vi "Gather_Deal_Data_BK.vi"(8 "strModelChoice":string(combo)="WD5500", 9 "写指令":bool=TRUE, 10 "VISA resource name":refnum<visa-resource-name>="COM1" caption="VISA资源名称") -> (2 "缓冲区数据":u32=284, 3 "strResultArrayOut":string[](array[string]))   [LabVIEW 2011]
uses:
  <vilib>/Instr/_visa.llb/VISA Configure Serial Port (Instr).vi
panel:
  out "mu08BufSize":u8
  out "mbfDealData":bool
  out "mu08SendCmd":u8=3
  in  "CmdNumCount":u8
  out "mu08ArrayBuf0":u8[](array[numeric])=[90, 165, 142, 1, 240, 0, 1, 88, 200, 2, 0, 207, 3, 0, 219, 7, 1, 40, 11, 0, 0, 12, 0, 0, 13, 0, 0, 14, 0, 0, 21, 0, 0, 22, 0, 0, 23, 0, 0, 24, 150, 154, 29, 0, 0, 0, 0, 31, 0, 0, 33, 0, 34, 1, 64, 35, 0, 41, 0, 42, 0, 43, 0, 44, 12, 158, 45, 0, 0, 46, 0, 240, 47, 240, 48, 0, 49, 0, 50, 136, 51, 0, 52, 0, 53, 0, 54, 132, 58, 0, 59, 0, 60, 241, 61, 32, 32, 32, 32, 82, 64, 73, 83, 90, 2, 4, 0, 2, 4, 0, 0, 0, 0, 2, 0, 0, 0, 104, 201, 113, 49, 49, 53, 202, 70, 52, 48, 53, 203, 57, 48, 48, 66, 204, 32, 32, 48, 53, 251, 6, 87, 112, 90, 165, 142, 1, 240, 0, 1, 88, 200, 2, 0, 207, 3, 0, 219, 7, 1, 40, 11, 0, 0, 12, 0, 0, 13, 0, 0, 14, 0, 0, 21, 0, 0, 22, 0, 0, 23, 0, 0, 24, 150, 151, 29, 0, 0, 0, 0, 31, 0, 0, 33, 0, 34, 1, 64, 35, 0, 41, 0, 42, 0, 43, 0, 44, 12, 158, 45, 0, 0, 46, 0, 240, 47, 240, 48, 0, 49, 0, 50, 136, 51, 0, 52, 0, 53, 0, 54, 132, 58, 0, 59, 0, 60, 241, 61, 32, 32, 32, 32, 82, 64, 73, 83, 90, 2, 4, 0, 2, 4, 0, 0, 0, 0, 2, 0, 0, 0, 104, 201, 113, 49, 49, 53, 202, 70, 52, 48, 53, 203, 57, 48, 48, 66, 204, 32, 32, 48, 53, 251, 6, 95, 118] format="0x%x"
  out "mu16ArrayBuf0":u16=284
  out "mu08ArrayDatas":u8[](array[numeric])=[90, 165, 142, 1, 240, 0, 1, 88, 200, 2, 0, 207, 3, 0, 219, 7, 1, 40, 11, 0, 0, 12, 0, 0, 13, 0, 0, 14, 0, 0, 21, 0, 0, 22, 0, 0, 23, 0, 0, 24, 150, 154, 29, 0, 0, 0, 0, 31, 0, 0, 33, 0, 34, 1, 64, 35, 0, 41, 0, 42, 0, 43, 0, 44, 12, 158, 45, 0, 0, 46, 0, 240, 47, 240, 48, 0, 49, 0, 50, 136, 51, 0, 52, 0, 53, 0, 54, 132, 58, 0, 59, 0, 60, 241, 61, 32, 32, 32, 32, 82, 64, 73, 83, 90, 2, 4, 0, 2, 4, 0, 0, 0, 0, 2, 0, 0, 0, 104, 201, 113, 49, 49, 53, 202, 70, 52, 48, 53, 203, 57, 48, 48, 66, 204, 32, 32, 48, 53, 251, 6, 87, 112] format="0x%x"
  out "mu08ArrayDatasSize":u16=142
  out "命令":string
  in  "mbfUartClearOne":bool=TRUE
  out "Time":u32=400
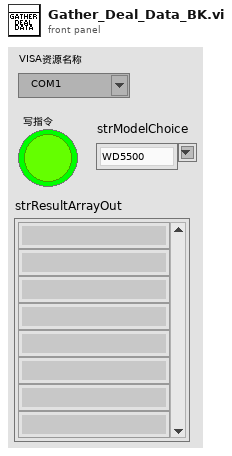
[diagram p1: front panel]
types:
  T1 = enum16{"open", "replace", "create", "open or create", "replace or create", "replace or create with confirmation"}
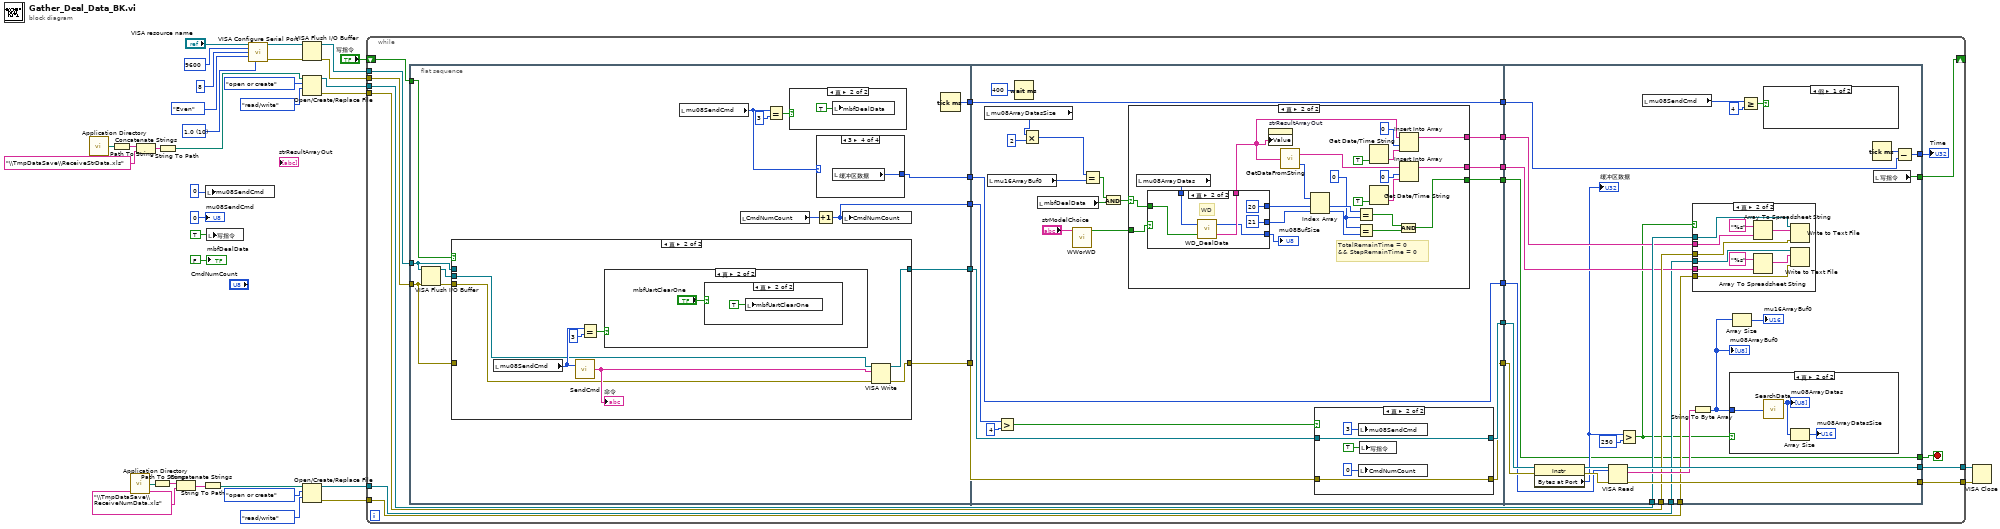
[diagram p0: block diagram]
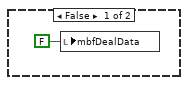
[diagram p2: hidden frame]
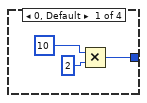
[diagram p3: hidden frame]
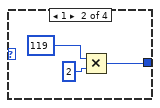
[diagram p4: hidden frame]
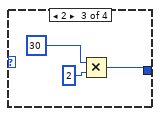
[diagram p5: hidden frame]
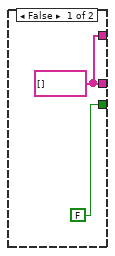
[diagram p9: hidden frame]
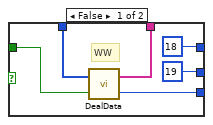
[diagram p10: hidden frame]
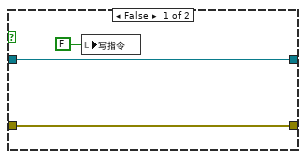
[diagram p11: hidden frame]
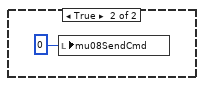
[diagram p14: hidden frame]
diagram:
  w30 = u16 10 items=["1.0"=10, "1.5"=15, "2.0"=20] ("stop bits (10: 1 bit)")
  n1 = call <vilib>:"Application Directory.vi"() -> ("Application Directory"=w8:path)
  n2 = Path To String(path=w8) -> (string=w7:string)
  n3 = call <vilib>:"Application Directory.vi"() -> ("Application Directory"=w4:path)
  n4 = Concatenate Strings(w7, "\\TmpDataSave\\ReceiveStrData.xls" ("字符串")) -> (w5:string)
  n5 = Path To String(path=w4) -> (string=w3:string)
  n6 = String To Path(string=w5) -> (path=w16:path)
  n7 = Concatenate Strings(w3, "\\TmpDataSave\\ReceiveNumData.xls" ("字符串")) -> (w1:string)
  n8 = String To Path(string=w1) -> (path=w9:path)
  n9 = local write "mu08SendCmd"(u8 0 ("Cmd值")) -> ()
  n10 = local write "写指令"(TRUE ("写指令")) -> ()
  n11 = call-poly "VISA Configure Serial Port"("VISA resource name"="VISA resource name", "baud rate (9600)"=u32 9600, "data bits (8)"=u16 8, "parity (0:none)"=enum16{"None", "Odd", "Even", "Mark", "Space"}."Even", "stop bits (10: 1 bit)"=w30) -> ("VISA resource name out"=w26:refnum<visa-resource-name>, "error out"=w25:errorcluster)  [unwired: 9 in]
  n12 = VISA Flush I/O Buffer(VISA resource name=w26, error in (no error)=w25) -> (VISA resource name out=w24:refnum<visa-resource-name>, error out=w23:errorcluster)  [unwired: 1 in]
  n13 = Open/Create/Replace File(file path (use dialog)=w16, operation (0:open)=T1."open or create" ("操作(0:open)"), access (0:read/write)=enum16{"read/write", "read-only", "write-only"}."read/write" ("权限(0:read/write)")) -> (refnum out=w15:refnum<file>, error out=w14:errorcluster)  [unwired: 3 in, 1 out]
  n14 = Open/Create/Replace File(file path (use dialog)=w9, operation (0:open)=T1."open or create" ("操作(0:open)"), access (0:read/write)=enum16{"read/write", "read-only", "write-only"}."read/write" ("权限(0:read/write)")) -> (refnum out=w12:refnum<file>, error out=w13:errorcluster)  [unwired: 3 in, 1 out]
  n15 = while {
    tunnel: w24 -> [w58]
    tunnel: w23 -> [w57]
    tunnel: [w54] -> w29
    tunnel: [w53] -> w28
    shift-right: [w51] -> _
    shift-left: "写指令" -> [w52]
    tunnel: w15 -> [w46]
    tunnel: w14 -> [w45]
    tunnel: w13 -> [w39]
    tunnel: w12 -> [w38]
    stop <- w36 stop-if-true
    n16 = flat-sequence {
      tunnel: w58 -> [w64]
      tunnel: w57 -> [w63]
      tunnel: [w72] -> w56
      tunnel: [w71] -> w55
      tunnel: w52 -> [w70]
      tunnel: [w68] -> w50
      tunnel: [w59] -> w47
      tunnel: [w60] -> w43
      tunnel: w56 -> [w112]
      tunnel: w55 -> [w111]
      tunnel: w50 -> [w115]
      tunnel: [w114] -> w49
      tunnel: [w113] -> w48
      tunnel: w47 -> [w99]
      tunnel: [w110] -> w44
      tunnel: w43 -> [w109]
      tunnel: [w109] -> w42
      tunnel: [w108] -> w40
      tunnel: [w103] -> w37
      tunnel: [w99] -> w35
      tunnel: w49 -> [w185]
      tunnel: w48 -> [w184]
      tunnel: [w188] -> w54
      tunnel: [w187] -> w53
      tunnel: [w179] -> w51
      tunnel: w46 -> [w177]
      tunnel: w45 -> [w176]
      tunnel: w44 -> [w175]
      tunnel: w42 -> [w173]
      tunnel: [w172] -> w41
      tunnel: w40 -> [w171]
      tunnel: w39 -> [w170]
      tunnel: w38 -> [w169]
      tunnel: [w164] -> w36
      tunnel: w37 -> [w164]
      tunnel: w35 -> [w180]
      frame #0 {
        n17 = VISA Flush I/O Buffer(VISA resource name=w64, error in (no error)=w63) -> (VISA resource name out=w61:refnum<visa-resource-name>, error out=w62:errorcluster)  [unwired: 1 in]
        n18 = case shown="真" w70 {
          tunnel: w64 -> [w86 _]
          tunnel: w63 -> [w85 _]
          tunnel: [w86 w94] -> w72
          tunnel: [w85 w93] -> w71
          tunnel: w62 -> [_ w88]
          tunnel: w61 -> [_ w87]
          frame False {
          }
          frame True {
            n19 = local read "mu08SendCmd"() -> (w90:u8)
            n20 = call "SendCmd.vi"("索引 (行)"=w90) -> ("字符串"=w92:string)  [unwired: 1 in]
            "命令" <- w92
            n21 = Equal?(x=w90, y=u8 3) -> (x = y?=w89:bool)
            n22 = case shown="真" w89 {
              frame False {
              }
              frame True {
                n23 = case shown="真" "mbfUartClearOne" {
                  frame False {
                  }
                  frame True {
                    n24 = local write "mbfUartClearOne"(TRUE ("mbfUartClearOne")) -> ()
                  }
                }
              }
            }
            n25 = VISA Write(VISA resource name=w87, write buffer=w92, error in (no error)=w88) -> (VISA resource name out=w94:refnum<visa-resource-name>, error out=w93:errorcluster)  [unwired: 1 out]
          }
        }
        n26 = local read "mu08SendCmd"() -> (w67:u8)
        n27 = local read "CmdNumCount"() -> (w69:u8)
        n28 = Equal?(x=w67, y=u8 3) -> (x = y?=w65:bool)
        n29 = case shown="真" w65 {
          frame False {
            n30 = local write "mbfDealData"(FALSE ("mbfDealData")) -> ()
          }
          frame True {
            n31 = local write "mbfDealData"(TRUE ("mbfDealData")) -> ()
          }
        }
        n32 = case shown="3" w67 {
          tunnel: [w75 w78 w81 w84] -> w59
          frame 0, Default {
            n33 = Multiply(x=10, y=2) -> (x*y=w75:i32)
          }
          frame 1 {
            n34 = Multiply(x=119, y=2) -> (x*y=w78:i32)
          }
          frame 2 {
            n35 = Multiply(x=30, y=2) -> (x*y=w81:i32)
          }
          frame 3 {
            n36 = local read "缓冲区数据"() -> (w84:u32)
          }
        }
        n37 = Increment(x=w69) -> (x+1=w68:u8)
        n38 = local write "CmdNumCount"(w68) -> ()
        n39 = Tick Count (ms)() -> (millisecond timer value=w60:u32)
      }
      frame #1 {
        n40 = local read "mu08ArrayDatasSize"() -> (w102:u16)
        n41 = local read "mu16ArrayBuf0"() -> (w107:u16)
        n42 = Greater?(x=w115, y=u8 4) -> (0:w116:bool)
        n43 = Wait (ms)(milliseconds to wait=u32 400 ("等待时间（毫秒）")) -> ()  [unwired: 1 out]
        n44 = Multiply(x=w102, y=u8 2) -> (x*y=w100:u16)
        n45 = local read "mbfDealData"() -> (w106:bool)
        n46 = call "WWorWD.vi"("strModelChoice"="strModelChoice") -> ("WWorWD"=w97:bool)  [unwired: 9 in, 1 out]
        n47 = Equal?(x=w100, y=w107) -> (x = y?=w105:bool)
        n48 = And(x=w105, y=w106) -> (x .and. y?=w104:bool)
        n49 = case shown="真" w104 {
          selector: w104 -> [_ w123]
          tunnel: [w120 w141] -> w110
          tunnel: [w120 w136] -> w108
          tunnel: [FALSE w128] -> w103
          tunnel: w97 -> [_ w124]
          frame False {
            w120 = string[] []
          }
          frame True {
            w132 = u32 0 ("y")
            # "TotalRemainTime = 0\n&& StepRemainTime = 0"
            n50 = local read "mu08ArrayDatas"() -> (w127:u8[])
            n51 = case shown="真" w124 {
              tunnel: [w149 w155] -> w121
              tunnel: [w148 w154] -> w122
              tunnel: w127 -> [w147 w153]
              tunnel: [18 ("索引") 20 ("索引")] -> w126
              tunnel: [19 ("索引") 21 ("索引")] -> w125
              tunnel: w123 -> [w144 w150]
              frame False {
                # "WW"
                n52 = call "DealData.vi"("mbfDealData"=w144, "ArrayIn"=w147) -> ("mu08BufSize"=w148:u8, "Result"=w149:string[])
              }
              frame True {
                # "WD"
                n53 = call "WD_DealData.vi"("mbfDealData"=w150, "ArrayIn"=w153) -> ("ResultArrayOut"=w155:string[], "mu08BufSize"=w154:u8)
              }
            }
            "mu08BufSize" <- w122
            n54 = property on="strResultArrayOut" class="Arr (严格)"("Value"=w121) -> ()  [unwired: 2 in, 2 out]
            n55 = call "GetDataFromString.vi"("strArrayIn"=w121) -> ("strArrayBuf"=w135:string[], "mu32ArrayOut"=w134:u32[])
            n56 = Index Array(array=w134, index #1=w126, index #2=w125) -> (element #1=w133:u32, element #2=w131:u32)
            n57 = Equal?(x=w133, y=w132) -> (x = y?=w130:bool)
            n58 = Equal?(x=w132, y=w131) -> (x = y?=w129:bool)
            n59 = Get Date/Time String(want seconds? (F)=TRUE ("需要秒？(F)")) -> (time string=w142:string)  [unwired: 2 in, 1 out]
            n60 = Get Date/Time String(want seconds? (F)=TRUE ("需要秒？(F)")) -> (time string=w138:string)  [unwired: 2 in, 1 out]
            n61 = And(x=w130, y=w129) -> (x .and. y?=w128:bool)
            n62 = Insert Into Array(array=w121, index=0 ("索引"), new element=w142) -> (w141:string[])
            n63 = Insert Into Array(array=w135, index=0 ("索引"), new element=w138) -> (w136:string[])
          }
        }
        n64 = case shown="真" w116 {
          tunnel: [w157 w161] -> w114
          tunnel: [w156 w160] -> w113
          tunnel: w112 -> [w157 w161]
          tunnel: w111 -> [w156 w160]
          frame False {
            n65 = local write "写指令"(FALSE ("写指令")) -> ()
          }
          frame True {
            n66 = local write "mu08SendCmd"(u8 3 ("mu08SendCmd")) -> ()
            n67 = local write "CmdNumCount"(u8 0 ("CmdNumCount")) -> ()
            n68 = local write "写指令"(TRUE ("写指令")) -> ()
          }
        }
      }
      frame #2 {
        n69 = property class="Instr"(reference=w185, error in=w184) -> (reference out=w190:refnum<visa-resource-name>, error out=w189:errorcluster, "Bytes at Port"=w167:u32)
        "缓冲区数据" <- w167
        n70 = VISA Read(VISA resource name=w190, byte count=w180, error in (no error)=w189) -> (VISA resource name out=w188:refnum<visa-resource-name>, read buffer=w186:string, error out=w187:errorcluster)  [unwired: 1 out]
        n71 = Greater?(x=w167, y=250) -> (0:w166:bool)
        n72 = local read "mu08SendCmd"() -> (w183:u8)
        n73 = case shown="真" w166 {
          tunnel: w177 -> [_ w201]
          tunnel: w176 -> [_ w200]
          tunnel: w175 -> [_ w199]
          tunnel: w171 -> [_ w198]
          tunnel: w170 -> [_ w195]
          tunnel: w169 -> [_ w194]
          frame False {
          }
          frame True {
            n74 = Array To Spreadsheet String(array=w199, 3:"%s" ("格式字符串")) -> (spreadsheet string=w203:string)  [unwired: 1 in]
            n75 = Array To Spreadsheet String(array=w198, 3:"%s" ("格式字符串")) -> (spreadsheet string=w196:string)  [unwired: 1 in]
            n76 = Write to Text File(file (use dialog)=w201, text=w203, error in=w200) -> ()  [unwired: 1 in, 3 out]
            n77 = Write to Text File(file (use dialog)=w194, text=w196, error in=w195) -> ()  [unwired: 1 in, 3 out]
          }
        }
        n78 = String To Byte Array(string=w186) -> (unsigned byte array=w165:u8[])
        "mu08ArrayBuf0" <- w165
        n79 = case shown="真" w166 {
          tunnel: w165 -> [_ w192]
          frame False {
          }
          frame True {
            n80 = call "SearchData.vi"("ArrayIn"=w192) -> ("ArrayOut"=w191:u8[])  [unwired: 2 out]
            "mu08ArrayDatas" <- w191
            n81 = Array Size(array=w191) -> (size(s)=→"mu08ArrayDatasSize":i32)
          }
        }
        n82 = Array Size(array=w165) -> (size(s)=→"mu16ArrayBuf0":i32)
        n83 = Greater Or Equal?(x=w183, y=u8 4) -> (x >= y?=w181:bool)
        n84 = case shown="假" w181 {
          frame False {
          }
          frame True {
            n85 = local write "mu08SendCmd"(u8 0 ("Cmd值")) -> ()
          }
        }
        n86 = Tick Count (ms)() -> (millisecond timer value=w174:u32)
        n87 = local read "写指令"() -> (w179:bool)
        n88 = Subtract(x=w174, y=w173) -> (x-y=w172:u32)
      }
    }
    "Time" <- w41
  }
  n89 = VISA Close(VISA resource name=w29, error in (no error)=w28) -> ()  [unwired: 1 out]
  "mu08SendCmd" <- u8 0 ("mu08SendCmd")
  "mbfDealData" <- FALSE ("mbfDealData")
